vi "Robot Main.vi"() -> ()   [LabVIEW 2011]
doc: "This VI imlements the framework and scheduler for your robotics program. It should not be necessary to modify the framework. You are expected to add your code to the VIs called from Robot Main, the ones located in the Team Code within the project."
uses:
  <vilib>/Rock Robotics/WPI/Camera/WPI_CameraImageSize.ctl
  Robot Global Data.vi
panel:
  out "Timings":cluster{"Call Name":string, "Delta (ms)":u32}[](array[cluster])
  in  "Image Size":T1=enum."320x240"
  in  "Enable Vision":bool
  in  "Finish":bool
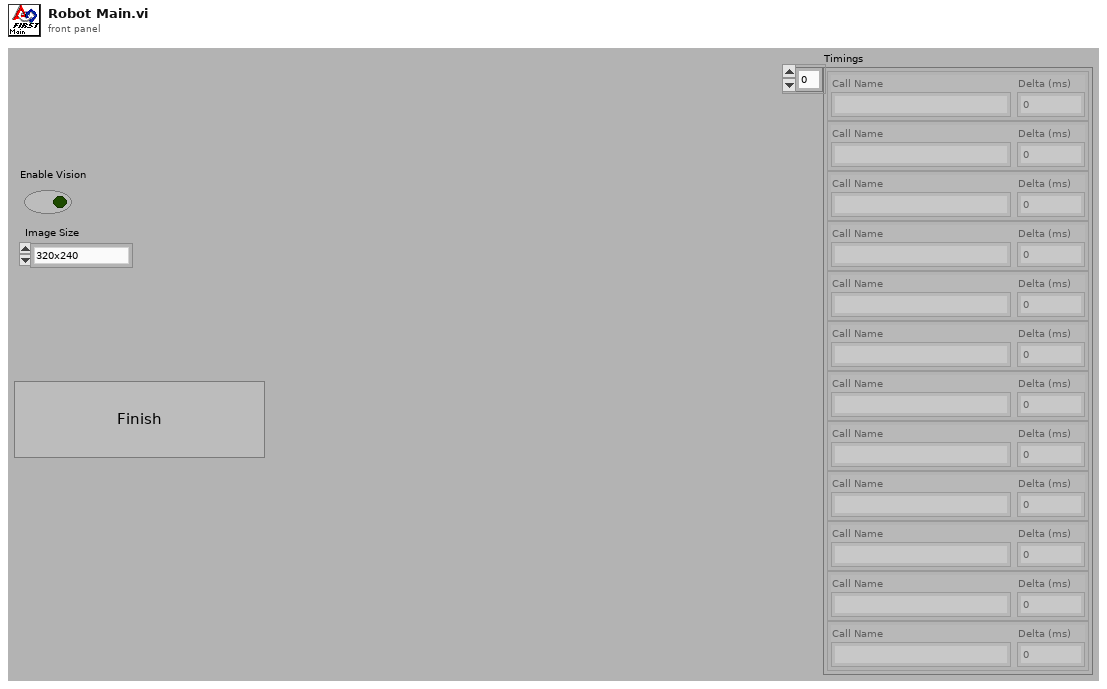
[diagram p1: front panel]
types:
  T1 = typedef "WPI_CameraImageSize.ctl" = enum16{"640x480", "320x240", "160x120"}
  T2 = typedef "WPI_DriverStationMatch Info.ctl" = cluster{"Autonomous Elapsed Seconds":dbl, "TeleOp Elapsed Seconds":dbl, "Disabled Elapsed Seconds":dbl, "Visited Autonomous":bool, "Visited TeleOp":bool, "Visited Disabled":bool, "Autonomous Settings":cluster{"Autonomous Style":enum16{"Iterative", "Independent"}, "VI Refnum":refnum<vi>}}
  T3 = typedef "WPI_DriverStationDerivedRobotMode.ctl" = enum16{"Init", "Execute", "Stop"}
  T4 = typedef "WPI_DriverStationRobotMode.ctl" = enum16{"Autonomous Disabled", "Autonomous Enabled", "Teleop Disabled", "Teleop Enabled", "Timeout", "Finish"}
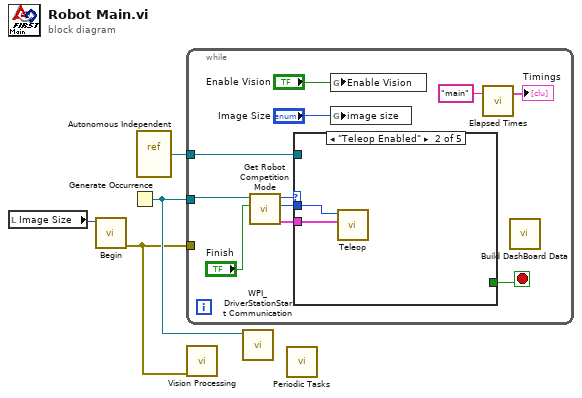
[diagram p0: block diagram]
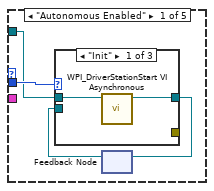
[diagram p2: hidden frame]
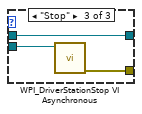
[diagram p4: hidden frame]
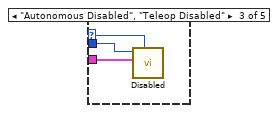
[diagram p5: hidden frame]
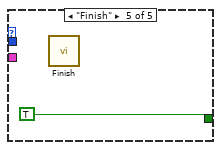
[diagram p7: hidden frame]
diagram:
  n1 = local read "Image Size"() -> (w3:T1)
  n2 = call "Begin.vi"("Image Size"=w3) -> ("error out"=w1:errorcluster)  [unwired: 10 out]
  n3 = Generate Occurrence() -> (w4:refnum<k4>)
  n4 = vi-ref "Autonomous Independent.vi"() -> (w2:refnum<vi>)
  n5 = while {
    tunnel: w4 -> [w13]
    tunnel: w1 -> [_]
    tunnel: w2 -> [w8]
    stop <- w10 stop-if-true
    n6 = call "Get Robot Competition Mode.vi"("Finish"="Finish", "DS Occurrence"=w13) -> ("Match Info out"=w11:T2, "Call Context"=w15:T3, "Robot Mode"=w14:T4)  [unwired: 7 out]
    n7 = case shown="\"Teleop Enabled\"" w14 {
      selector: w14 -> [_ _ w28 _ _]
      tunnel: w15 -> [w19 w27 w30 _ _]
      tunnel: w11 -> [_ w26 w29 _ _]
      tunnel: [_ _ _ _ TRUE] -> w10
      tunnel: w8 -> [w18 _ _ _ _]
      frame "Autonomous Enabled" {
        n8 = feedback #1() -> (w16:refnum<vi>)  [unwired: 1 out]
        n9 = case shown="\"Init\"" w19 {
          tunnel: w18 -> [w21 _ w24]
          tunnel: [w20 w22 w24] -> w17
          tunnel: w16 -> [_ w22 w25]
          tunnel: [_ _ w23] -> _
          frame "Init" {
            n10 = call <vilib>:"WPI_DriverStationStart VI Asynchronous.vi"("VI"=w21) -> ("VI out"=w20:refnum<vi>)  [unwired: 10 out]
          }
          frame "Execute", Default {
            # "Nothing to do"
          }
          frame "Stop" {
            n11 = call <vilib>:"WPI_DriverStationStop VI Asynchronous.vi"("VI Refnum"=w25) -> ("error out"=w23:errorcluster)  [unwired: 10 out]
          }
        }
        n12 = feedback-in #1(w17) -> ()
      }
      frame "Teleop Enabled" {
        n13 = call "Teleop.vi"("Match Info"=w26, "Call Context"=w27) -> ()  [unwired: 1 in, 9 out]
      }
      frame "Autonomous Disabled", "Teleop Disabled" {
        n14 = call "Disabled.vi"("Robot Mode"=w28, "Match Info"=w29, "Call Context"=w30) -> ()  [unwired: 1 in, 8 out]
      }
      frame "Timeout" {
      }
      frame "Finish" {
        n15 = call "Finish.vi"() -> ()  [unwired: 1 in, 7 out]
      }
    }
    n16 = global write "Robot Global Data.vi" "Enable Vision"("Enable Vision") -> ()
    n17 = global write "Robot Global Data.vi" "image size"("Image Size") -> ()
    n18 = call "Elapsed Times.vi"("Call Name"="main") -> ("Timings"=→"Timings":cluster{"Call Name":string, "Delta (ms)":u32}[])  [unwired: 2 in]
    n19 = call "Build DashBoard Data.vi"() -> ()  [unwired: 1 in, 11 out]
  }
  n20 = call "Vision Processing.vi"("error in (no error)"=w1) -> ()  [unwired: 1 in, 6 out]
  n21 = call <vilib>:"WPI_DriverStationStart Communication.vi"("occurrence"=w4) -> ()  [unwired: 11 out]
  n22 = call "Periodic Tasks.vi"() -> ()  [unwired: 2 in, 10 out]
